vi "Check QDFunction Has Shortcut.vi"(8 "error in (no error)":errorcluster, 9 "QDShortcut":string, 10 "QDFullName":string, 11 "QDDialogList in":refnum<class "QDDialogList.lvclass">) -> (0 "error out":errorcluster, 2 "HasShortcut(False)":bool, 3 "QDDialogList out":refnum<class "QDDialogList.lvclass">)   [LabVIEW 2015, in "QDDialogList.lvclass"]
uses:
  QDDialogList.lvclass
  QDDialogList.lvclass/QDDialogList.ctl
  <vilib>/Utility/error.llb/Error Cluster From Error Code.vi
  <vilib>/ErrorRing/Error Ring.xnode
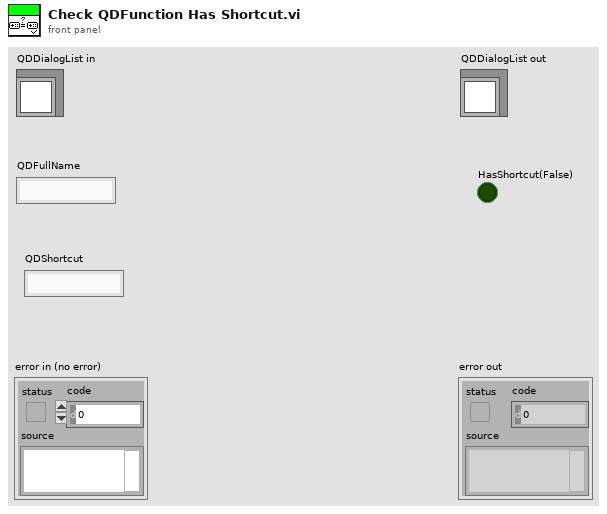
[diagram p1: front panel]
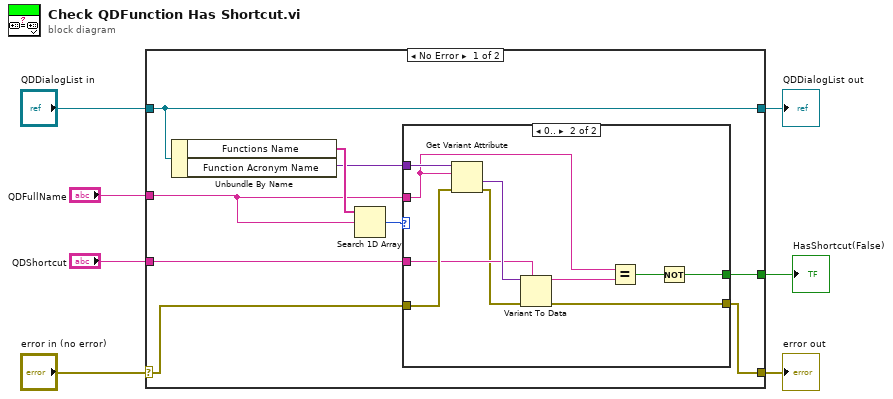
[diagram p0: block diagram]
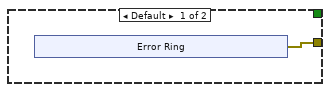
[diagram p2: hidden frame]
diagram:
  n1 = case shown="No Error" "error in (no error)" {
    selector: "error in (no error)" -> [w10 w34]
    tunnel: [w8 w34] -> w6
    tunnel: [w16 w33] -> w4
    tunnel: "QDDialogList in" -> [w16 w33]
    tunnel: "QDFullName" -> [w13 _]
    tunnel: "QDShortcut" -> [w12 _]
    tunnel: [w9 _] -> w1
    frame No Error {
      n2 = Unbundle By Name(w16) -> ("Functions Name"=w15:string[], "Function Acronym Name"=w11:variant)
      n3 = Search 1D Array(1D array=w15, element=w13) -> (index of element=w14:i32)  [unwired: 1 in]
      n4 = case shown="0.." w14 {
        tunnel: w13 -> [_ w26]
        tunnel: w12 -> [_ w29]
        tunnel: [w17 w25] -> w8
        tunnel: w11 -> [_ w32]
        tunnel: w10 -> [_ w31]
        tunnel: [_ w23] -> w9
        frame Default {
          n5 = xnode "Error Ring"() -> ("error out"=w17:errorcluster)
        }
        frame 0.. {
          n6 = Get Variant Attribute(Variant=w32, name=w26, error in=w31) -> (value=w30:variant, error out=w28:errorcluster)  [unwired: 1 in, 2 out]
          n7 = Variant To Data(error in=w28, type=w29, Variant=w30) -> (data=w27:string, error out=w25:errorcluster)
          n8 = Equal?(x=w26, y=w27) -> (x = y?=w24:bool)
          n9 = Not(x=w24) -> (.not. x?=w23:bool)
        }
      }
    }
    frame Error {
    }
  }
  "error out" <- w6
  "QDDialogList out" <- w4
  "HasShortcut(False)" <- w1
